vi "FUG_MagnetPS.ProcCases.vi"(0 "i ref in":refnum<vi>, 1 "selector":string, 2 "Data":T1, 3 "call cluster":T2={"Object"="", "Selector"="", "CallType"=enum."synchronous", "Async Object"="", "Async Selector"="", "Data Descriptor"="", "Data"=[], "Error #"=0, "Expire"=0}, 5 "error in (no error)":errorcluster) -> (14 "i ref out":refnum<vi>, 17 "answer cluster":T2={"Object"="", "Selector"="", "CallType"=enum."synchronous", "Async Object"="", "Async Selector"="", "Data Descriptor"="", "Data"=[], "Error #"=0, "Expire"=0}, 19 "error out":errorcluster)   [LabVIEW 2014, in "FUG_MagnetPS.lvlib"]
doc: "This method is called by a process from within the default case in the event loop. The methods of a class that are linked to events will be called from THIS method. Add your code here."
uses:
  FUG_MagnetPS.lvlib
  CS_Core/CSSystem/CoreDefs/CoreDefs.call_type.ctl
  CS_Core/BaseProcess/BaseProcess.descriptor string definition.ctl
  CS_Core/CSSystem/CoreDefs/CoreDefs.rawDataType.ctl
  CS_Core/CSSystem/CoreLib/CoreLib.string 2 byte array.vi
  CS_Core/CSSystem/CoreLib/CoreLib.byte array 2 short.vi
  CS_Core/CSSystem/CoreLib/CoreLib.byte array 2 double.vi
  CS_Core/CSSystem/CoreLib/CoreLib.double 2 byte array.vi
  CS_Core/CSSystem/CoreLib/CoreLib.lvlib
  CS_Core/BaseProcess/BaseProcess.lvlib
  CS_PowerSupply/FUG_PowerSupply/FUG_PowerSupply.lvlib
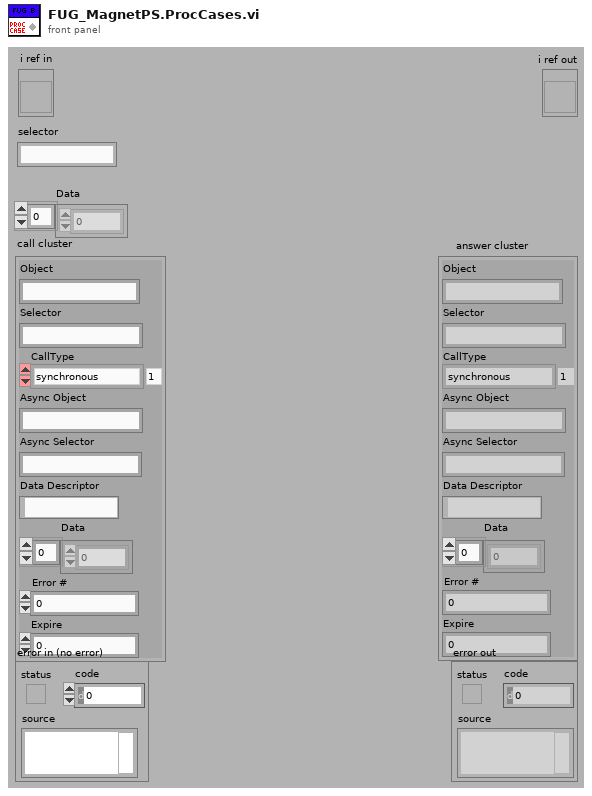
[diagram p1: front panel]
types:
  T1 = typedef "CoreDefs.rawDataType.ctl" = i8[]
  T2 = typedef "CoreDefs.call_type.ctl" = cluster{"Object":string, "Selector":string, "CallType":enum16{"simple", "synchronous", "asynchronous"}, "Async Object":string, "Async Selector":string, "Data Descriptor":T3, "Data":T1, "Error #":i32, "Expire":u32}
  T3 = typedef "BaseProcess.lvlib/BaseProcess.descriptor string definition.ctl" = string
  T4 = typedef "FUG_MagnetPS.lvlib/FUG_MagnetPS.i attribute.ctl" = cluster{"Gaussmeter":string, "SetField":dbl, "MagneticField queue":refnum<queue>, "Field Callback ID":i32, "nomCurrent":dbl, "Proportional":dbl, "Regulation?":bool, "actFieldID":i32, "nomFieldID":i32, "nomAutoCurrentID":i32, "regCurrentID":i32}
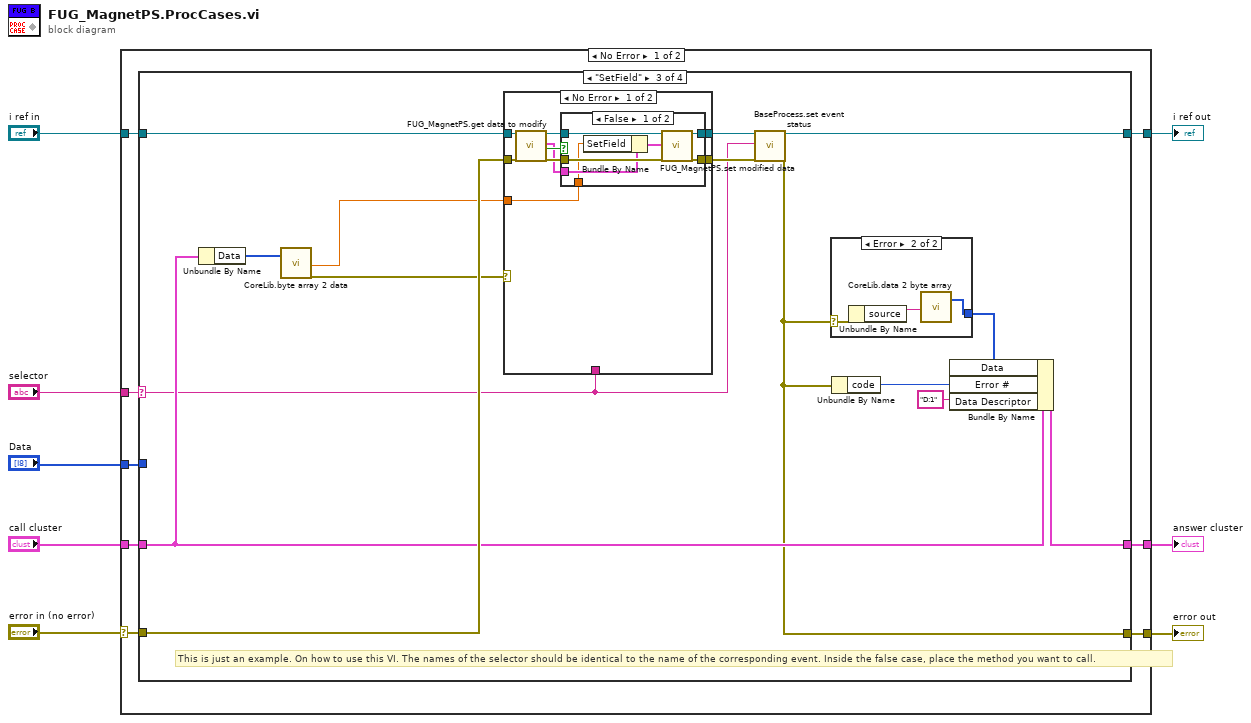
[diagram p0: block diagram]
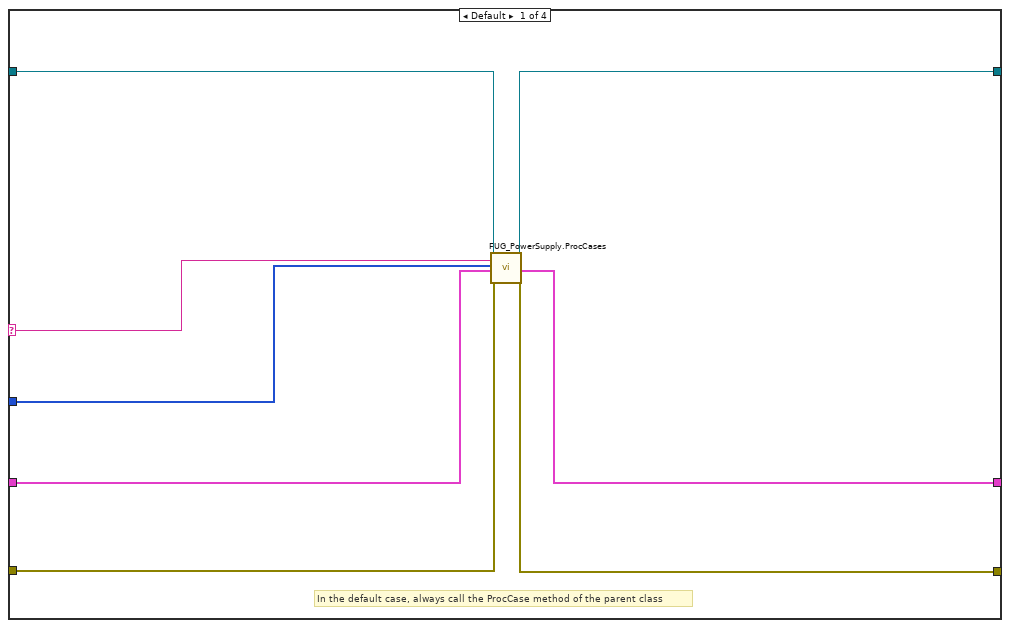
[diagram p2: hidden frame]
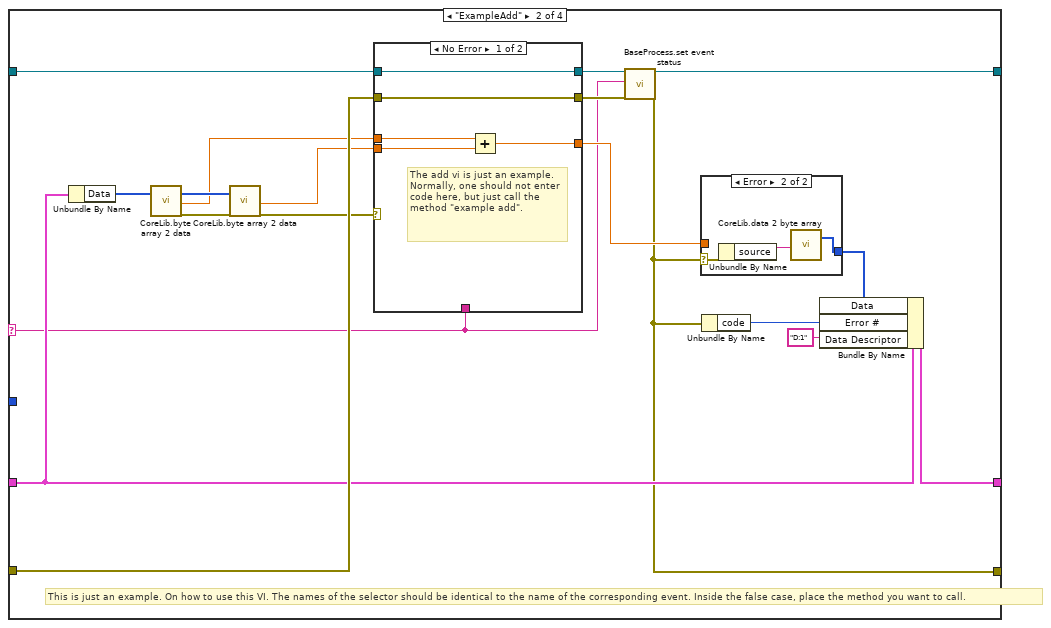
[diagram p3: hidden frame]
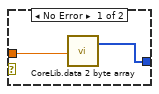
[diagram p4: hidden frame]
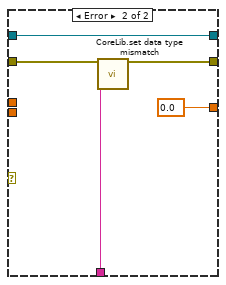
[diagram p5: hidden frame]
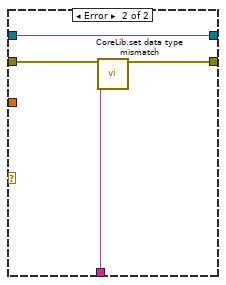
[diagram p8: hidden frame]
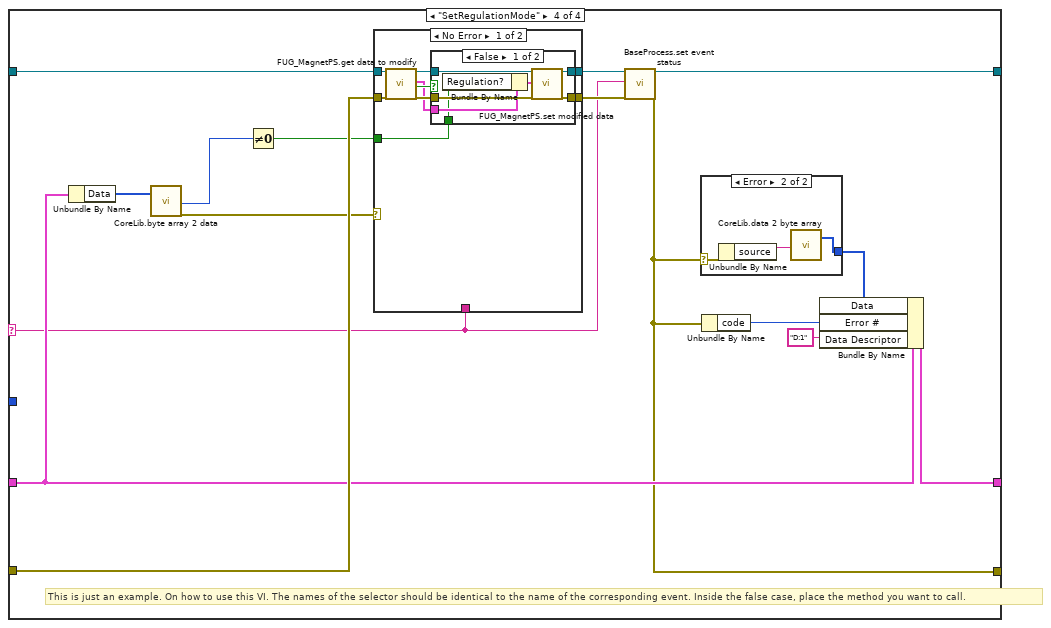
[diagram p9: hidden frame]
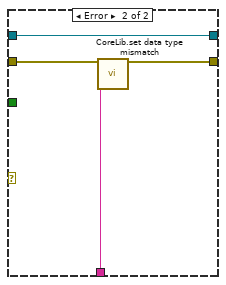
[diagram p12: hidden frame]
diagram:
  n1 = case shown="No Error" "error in (no error)" {
    selector: "error in (no error)" -> [w9 w140]
    tunnel: "selector" -> [w16 _]
    tunnel: [w15 w141] -> w7
    tunnel: "Data" -> [w14 _]
    tunnel: "call cluster" -> [w13 w141]
    tunnel: "i ref in" -> [w12 w142]
    tunnel: [w11 w142] -> w3
    tunnel: [w10 w140] -> w2
    frame No Error {
      n2 = case shown="\"SetField\"" w16 {
        selector: w16 -> [w18 w33 w64 w105]
        tunnel: w14 -> [w19 _ _ _]
        tunnel: w12 -> [w17 w43 w73 w114]
        tunnel: [w24 w32 w63 w104] -> w11
        tunnel: w13 -> [w20 w39 w70 w111]
        tunnel: [w21 w38 w69 w110] -> w15
        tunnel: w9 -> [w23 w42 w72 w113]
        tunnel: [w22 w34 w65 w106] -> w10
        frame Default {
          # "In the default case, always call the ProcCase method of the parent class"
          n3 = call "FUG_PowerSupply.ProcCases.vi"("i ref in"=w17, "selector"=w18, "Data"=w19, "call cluster"=w20, "error in (no error)"=w23) -> ("i ref out"=w24:refnum<vi>, "answer cluster"=w21:T2, "error out"=w22:errorcluster)  [unwired: 12 in]
        }
        frame "ExampleAdd" {
          # "This is just an example. On how to use this VI. The names of the selector should be identical to the name of the corresponding event. Inside the false case, place the method you want to call."
          n4 = Unbundle By Name(w39) -> ("Data"=w30:T1)
          n5 = call-poly "CoreLib.byte array 2 data.vi"("byteArray"=w30) -> ("byteArray out"=w29:T1, "d64"=w26:dbl, "error out"=w28:errorcluster)  [unwired: 16 in]
          n6 = call-poly "CoreLib.byte array 2 data.vi"("byteArray"=w29, "error in (no error)"=w28) -> ("d64"=w25:dbl, "error out"=w27:errorcluster)  [unwired: 15 in, 1 out]
          n7 = case shown="No Error" w27 {
            tunnel: [w50 w58] -> w36
            tunnel: w43 -> [w50 w58]
            tunnel: w42 -> [w51 w57]
            tunnel: [w51 w56] -> w35
            tunnel: w25 -> [w53 _]
            tunnel: [w52 0.0] -> w41
            tunnel: w33 -> [_ w54]
            tunnel: w26 -> [w49 _]
            frame No Error {
              # "The add vi is just an example. Normally, one should not enter code here, but just call the method \"example add\"."
              n8 = Add(x=w49, y=w53) -> (x+y=w52:dbl)
            }
            frame Error {
              n9 = call "CoreLib.set data type mismatch.vi"("error in (no error)"=w57, "error source"=w54) -> ("error out"=w56:errorcluster)  [unwired: 17 in]
            }
          }
          n10 = call "BaseProcess.set event status.vi"("i ref in"=w36, "EventStatus"=w33, "error in (no error)"=w35) -> ("i ref out"=w32:refnum<vi>, "error out"=w34:errorcluster)  [unwired: 14 in, 1 out]
          n11 = case shown="Error" w34 {
            selector: w34 -> [_ w48]
            tunnel: [w44 w46] -> w37
            tunnel: w41 -> [w45 _]
            frame No Error {
              n12 = call-poly "CoreLib.data 2 byte array.vi"("f64"=w45) -> ("byteArray out"=w44:T1)  [unwired: 18 in]
            }
            frame Error {
              n13 = Unbundle By Name(w48) -> ("source"=w47:string)
              n14 = call-poly "CoreLib.data 2 byte array.vi"("string"=w47) -> ("byteArray out"=w46:T1)  [unwired: 18 in]
            }
          }
          n15 = Unbundle By Name(w34) -> ("code"=w40:i32)
          n16 = Bundle By Name(cluster=w39, "Data"=w37, "Error #"=w40, "Data Descriptor"="D:1") -> (w38:T2)
        }
        frame "SetField" {
          # "This is just an example. On how to use this VI. The names of the selector should be identical to the name of the corresponding event. Inside the false case, place the method you want to call."
          n17 = Unbundle By Name(w70) -> ("Data"=w61:T1)
          n18 = call-poly "CoreLib.byte array 2 data.vi"("byteArray"=w61) -> ("d64"=w60:dbl, "error out"=w59:errorcluster)  [unwired: 16 in, 1 out]
          n19 = case shown="No Error" w59 {
            tunnel: [w82 w98] -> w67
            tunnel: w73 -> [w85 w98]
            tunnel: w72 -> [w84 w97]
            tunnel: [w80 w96] -> w66
            tunnel: w64 -> [_ w95]
            tunnel: w60 -> [w77 _]
            frame No Error {
              n20 = call "FUG_MagnetPS.get data to modify.vi"("i ref in"=w85, "error in (no error)"=w84) -> ("i ref out"=w83:refnum<vi>, "i attribute"=w78:T4, "timed out"=w79:bool, "error out"=w81:errorcluster)  [unwired: 14 in]
              n21 = case shown="False" w79 {
                tunnel: w83 -> [w92 w94]
                tunnel: [w91 w94] -> w82
                tunnel: w81 -> [w90 w93]
                tunnel: [w89 w93] -> w80
                tunnel: w78 -> [w88 _]
                tunnel: w77 -> [w86 _]
                frame False {
                  n22 = Bundle By Name(cluster=w88, "SetField"=w86) -> (w87:T4)
                  n23 = call "FUG_MagnetPS.set modified data.vi"("i ref in"=w92, "i attribute"=w87, "error in (no error)"=w90) -> ("i ref out"=w91:refnum<vi>, "error out"=w89:errorcluster)  [unwired: 15 in]
                }
                frame True {
                }
              }
            }
            frame Error {
              n24 = call "CoreLib.set data type mismatch.vi"("error in (no error)"=w97, "error source"=w95) -> ("error out"=w96:errorcluster)  [unwired: 17 in]
            }
          }
          n25 = call "BaseProcess.set event status.vi"("i ref in"=w67, "EventStatus"=w64, "error in (no error)"=w66) -> ("i ref out"=w63:refnum<vi>, "error out"=w65:errorcluster)  [unwired: 14 in, 1 out]
          n26 = case shown="Error" w65 {
            selector: w65 -> [_ w76]
            tunnel: [_ w74] -> w68
            frame No Error {
            }
            frame Error {
              n27 = Unbundle By Name(w76) -> ("source"=w75:string)
              n28 = call-poly "CoreLib.data 2 byte array.vi"("string"=w75) -> ("byteArray out"=w74:T1)  [unwired: 18 in]
            }
          }
          n29 = Unbundle By Name(w65) -> ("code"=w71:i32)
          n30 = Bundle By Name(cluster=w70, "Data"=w68, "Error #"=w71, "Data Descriptor"="D:1") -> (w69:T2)
        }
        frame "SetRegulationMode" {
          # "This is just an example. On how to use this VI. The names of the selector should be identical to the name of the corresponding event. Inside the false case, place the method you want to call."
          n31 = Unbundle By Name(w111) -> ("Data"=w102:T1)
          n32 = call-poly "CoreLib.byte array 2 data.vi"("byteArray"=w102) -> ("i16"=w100:i16, "error out"=w101:errorcluster)  [unwired: 16 in, 1 out]
          n33 = Not Equal To 0?(x=w100) -> (x != 0?=w99:bool)
          n34 = case shown="No Error" w101 {
            tunnel: [w123 w139] -> w108
            tunnel: w114 -> [w126 w139]
            tunnel: w113 -> [w125 w138]
            tunnel: [w121 w137] -> w107
            tunnel: w105 -> [_ w136]
            tunnel: w99 -> [w118 _]
            frame No Error {
              n35 = call "FUG_MagnetPS.get data to modify.vi"("i ref in"=w126, "error in (no error)"=w125) -> ("i ref out"=w124:refnum<vi>, "i attribute"=w119:T4, "timed out"=w120:bool, "error out"=w122:errorcluster)  [unwired: 14 in]
              n36 = case shown="False" w120 {
                tunnel: w124 -> [w133 w135]
                tunnel: [w132 w135] -> w123
                tunnel: w122 -> [w131 w134]
                tunnel: [w130 w134] -> w121
                tunnel: w119 -> [w129 _]
                tunnel: w118 -> [w127 _]
                frame False {
                  n37 = Bundle By Name(cluster=w129, "Regulation?"=w127) -> (w128:T4)
                  n38 = call "FUG_MagnetPS.set modified data.vi"("i ref in"=w133, "i attribute"=w128, "error in (no error)"=w131) -> ("i ref out"=w132:refnum<vi>, "error out"=w130:errorcluster)  [unwired: 15 in]
                }
                frame True {
                }
              }
            }
            frame Error {
              n39 = call "CoreLib.set data type mismatch.vi"("error in (no error)"=w138, "error source"=w136) -> ("error out"=w137:errorcluster)  [unwired: 17 in]
            }
          }
          n40 = call "BaseProcess.set event status.vi"("i ref in"=w108, "EventStatus"=w105, "error in (no error)"=w107) -> ("i ref out"=w104:refnum<vi>, "error out"=w106:errorcluster)  [unwired: 14 in, 1 out]
          n41 = case shown="Error" w106 {
            selector: w106 -> [_ w117]
            tunnel: [_ w115] -> w109
            frame No Error {
            }
            frame Error {
              n42 = Unbundle By Name(w117) -> ("source"=w116:string)
              n43 = call-poly "CoreLib.data 2 byte array.vi"("string"=w116) -> ("byteArray out"=w115:T1)  [unwired: 18 in]
            }
          }
          n44 = Unbundle By Name(w106) -> ("code"=w112:i32)
          n45 = Bundle By Name(cluster=w111, "Data"=w109, "Error #"=w112, "Data Descriptor"="D:1") -> (w110:T2)
        }
      }
    }
    frame Error {
    }
  }
  "answer cluster" <- w7
  "i ref out" <- w3
  "error out" <- w2
